vi "ThermalCond.vi"() -> ()   [LabVIEW 2014]
uses:
  Instance           2 23Saved   Vvstime-new-new .vi
  Instance           3 23Saved   Vvstime-new-new .vi
panel:
  out "XY Graph 4":cluster{dbl[], dbl[]}(graph)
  out "XY Graph 3":cluster{dbl[], dbl[]}(graph)
  in  "Voltmeter 1 address":string="22"
  in  "Wait (s)":dbl=3.0 format="%.2f"
  in  "Start/Stop":bool=TRUE
  in  "File Name":string="testing"
  # "Thermal Conductivity"
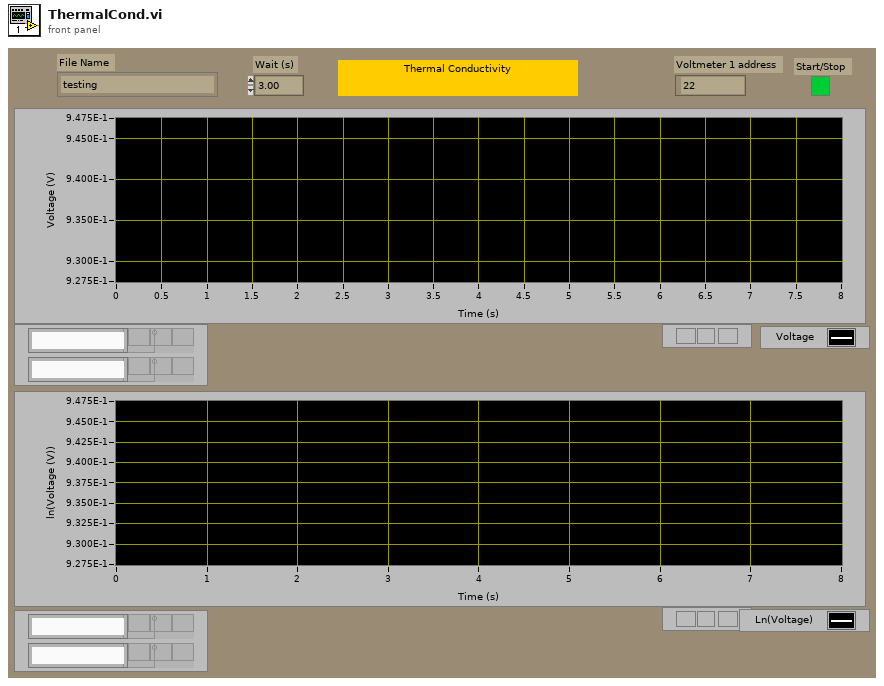
[diagram p1: front panel]
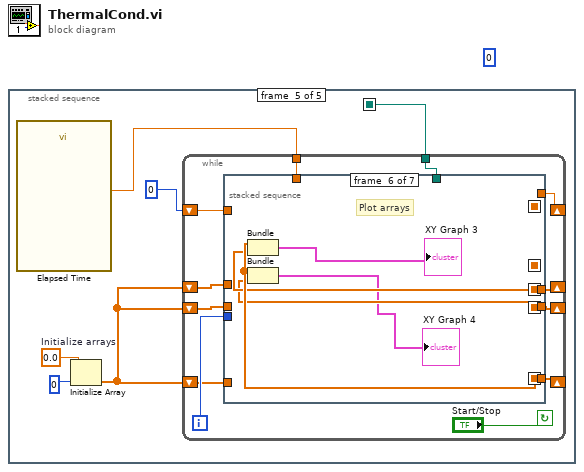
[diagram p0: block diagram]
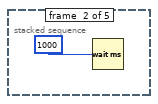
[diagram p3: hidden frame]
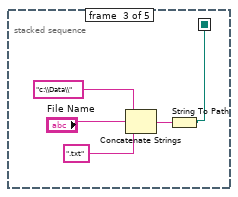
[diagram p4: hidden frame]
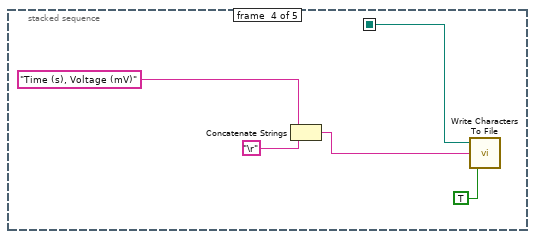
[diagram p5: hidden frame]
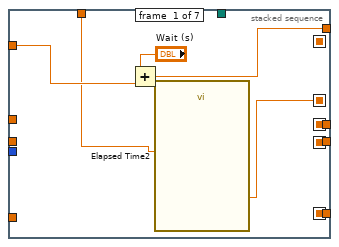
[diagram p6: hidden frame]
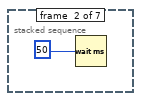
[diagram p7: hidden frame]
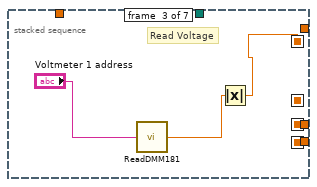
[diagram p8: hidden frame]
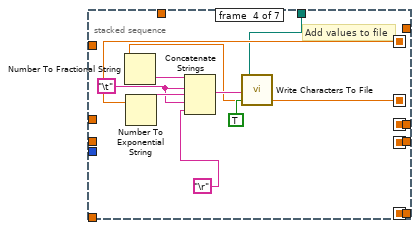
[diagram p9: hidden frame]
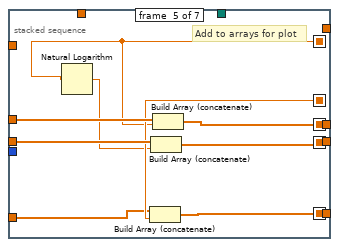
[diagram p10: hidden frame]
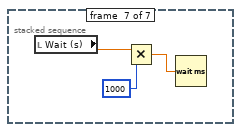
[diagram p11: hidden frame]
diagram:
  (unwired) 0
  n1 = stacked-sequence {
    seq-local: [_ _ w2 _ _] -> [_ _ _ w7 w14]
    frame #0 {
      # "init devices"
    }
    frame #1 {
      n2 = Wait (ms)(milliseconds to wait=1000) -> ()  [unwired: 1 out]
    }
    frame #2 {
      n3 = Concatenate Strings("c:\\Data\\", "File Name", ".txt") -> (w3:string)
      n4 = String To Path(string=w3) -> (path=w2:path)
    }
    frame #3 {
      n5 = Concatenate Strings("Time (s), Voltage (mV)", "\r") -> (w8:string)
      n6 = call <vilib>:"Write Characters To File.vi"("append to file? (new file:F)"=TRUE, "character string"=w8, "file path (dialog if empty)"=w7) -> ()  [unwired: 2 in, 1 out]
    }
    frame #4 {
      w17 = 0.0  # Initialize arrays
      n7 = call "Elapsed Time"() -> ("Get Start Time (s)"=w12:dbl)  [unwired: 12 in, 7 out]
      n8 = Initialize Array(w17, 0) -> (w15:dbl[])
      n9 = while {
        tunnel: w14 -> [w20]
        shift-left: 0 -> [w22]
        shift-right: [w21] -> _
        shift-left: w15 -> [w24]
        shift-right: [w23] -> _
        shift-left: w15 -> [w28]
        shift-right: [w18] -> _
        shift-left: w15 -> [w29]
        shift-right: [w27] -> _
        tunnel: w12 -> [w19]
        i -> [w25]
        stop <- "Start/Stop" continue-if-true
        n10 = stacked-sequence {
          seq-local: [w31 _ _ _ _ _ _] -> [_ _ _ w44 w52 _ _]
          seq-local: [_ _ _ _ w54 _ _] -> [_ _ _ _ _ w60 _]
          seq-local: [_ _ _ _ w53 _ _] -> [_ _ _ _ _ w59 _]
          seq-local: [_ _ w36 _ _ _ _] -> [_ _ _ w43 w48 _ _]
          seq-local: [_ _ _ _ w50 _ _] -> [_ _ _ _ _ w61 _]
          tunnel: w29 -> [_ _ _ _ w56 _ _]
          tunnel: w28 -> [_ _ _ _ w55 _ _]
          tunnel: [_ _ _ _ w54 _ _] -> w27
          tunnel: [_ _ _ _ w53 _ _] -> w18
          tunnel: w25 -> [_ _ _ _ _ _ _]
          tunnel: w22 -> [w32 _ _ _ _ _ _]
          tunnel: [w34 _ _ _ _ _ _] -> w21
          tunnel: w24 -> [_ _ _ _ w51 _ _]
          tunnel: [_ _ _ _ w50 _ _] -> w23
          tunnel: w20 -> [_ _ _ w40 _ _ _]
          tunnel: w19 -> [w30 _ _ _ _ _ _]
          frame #0 {
            n11 = Add(x="Wait (s)", y=w32) -> (x+y=w34:dbl)
            n12 = call "Elapsed Time2"("Set Start Time (s)"=w30) -> ("Elapsed Time (s)"=w31:dbl)  [unwired: 11 in, 7 out]
          }
          frame #1 {
            n13 = Wait (ms)(milliseconds to wait=50) -> ()  [unwired: 1 out]
          }
          frame #2 {
            # "Read Voltage"
            n14 = call "ReadDMM181.vi"("DMM GPIB Address"="Voltmeter 1 address") -> ("DMM read (mV)"=w37:dbl)
            n15 = Absolute Value(x=w37) -> (abs(x)=w36:dbl)
          }
          frame #3 {
            w41 = "\t"
            # "Add values to file"
            n16 = Number To Fractional String(number=w44) -> (F-format string=w47:string)  [unwired: 3 in]
            n17 = Number To Exponential String(number=w43) -> (E-format string=w42:string)  [unwired: 3 in]
            n18 = Concatenate Strings(w47, w41, w42, w41, "\r") -> (w45:string)
            n19 = call <vilib>:"Write Characters To File.vi"("append to file? (new file:F)"=TRUE, "character string"=w45, "file path (dialog if empty)"=w40) -> ()  [unwired: 2 in, 1 out]
          }
          frame #4 {
            # "Add to arrays for plot"
            n20 = Natural Logarithm(1:w48) -> (0:w49:dbl)
            n21 = Build Array (concatenate)(w51, w52) -> (w50:dbl[])
            n22 = Build Array (concatenate)(w55, w49) -> (w53:dbl[])
            n23 = Build Array (concatenate)(w56, w48) -> (w54:dbl[])
          }
          frame #5 {
            # "Plot arrays"
            n24 = Bundle(w61, w60) -> (→"XY Graph 3":cluster{dbl[], dbl[]})  [unwired: 1 in]
            n25 = Bundle(w61, w59) -> (→"XY Graph 4":cluster{dbl[], dbl[]})  [unwired: 1 in]
          }
          frame #6 {
            n26 = local read "Wait (s)"() -> (w62:dbl)
            n27 = Multiply(x=w62, y=1000) -> (x*y=w63:dbl)
            n28 = Wait (ms)(milliseconds to wait=w63) -> ()  [unwired: 1 out]
          }
        }
      }
    }
  }
